vi "interp type 2 1D.vi"(1 "NaN":dbl[](array[numeric]) format="%.2f") -> (0 "Interpolated":dbl[](array[numeric]) format="%.2f")   [LabVIEW 2016, in "comm.lvlib"]
uses:
  comm.lvlib
  <vilib>/Analysis/1siggen.llb/Ramp Pattern by Samples.vi
  <vilib>/Analysis/NI_AALBase.lvlib
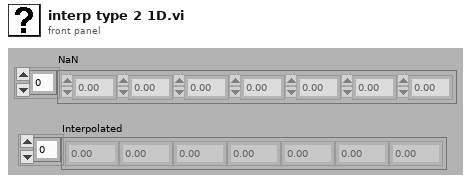
[diagram p1: front panel]
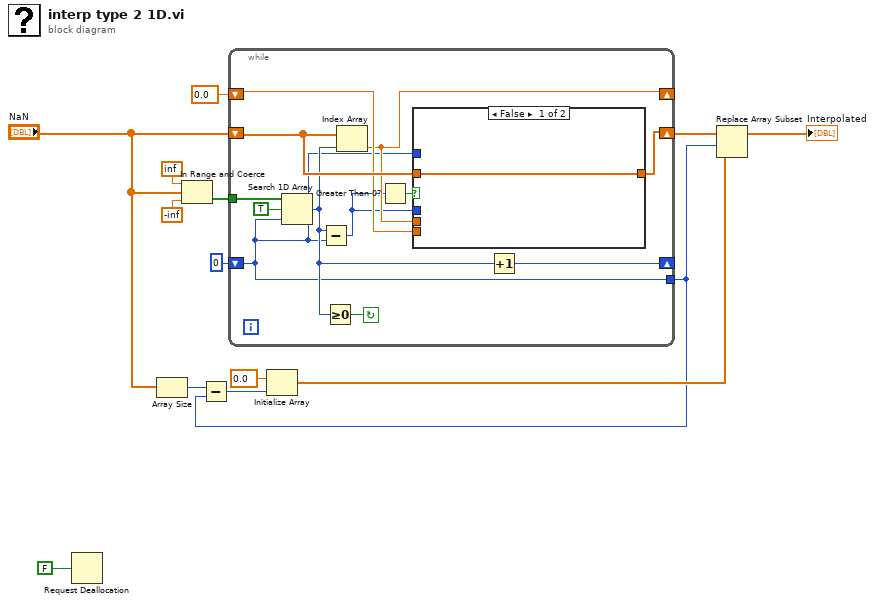
[diagram p0: block diagram]
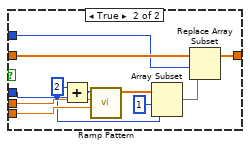
[diagram p2: hidden frame]
diagram:
  n1 = Request Deallocation(FALSE ("flag")) -> ()
  n2 = Array Size(array="NaN") -> (size(s)=w6:i32)
  n3 = In Range and Coerce(upper limit=inf, x="NaN", lower limit=-inf) -> (In Range?=w9:bool[])  [unwired: 1 out]
  n4 = while {
    tunnel: w9 -> [w26]
    shift-right: [w16] -> _
    shift-left: 0 -> [w15]
    shift-right: [w21] -> w3
    shift-left: "NaN" -> [w24]
    shift-right: [w22] -> _
    shift-left: 0.0 ("Numeric") -> [w23]
    tunnel: [w15] -> w1
    stop <- w19 continue-if-true
    n5 = Search 1D Array(1D array=w26, element=TRUE, start index (0)=w15) -> (index of element=w20:i32)
    n6 = Subtract(x=w20, y=w15) -> (x-y=w17:i32)
    n7 = Greater Or Equal To 0?(x=w20) -> (x >= 0?=w19:bool)
    n8 = Index Array(array=w24, index=w20) -> (element=w22:dbl)
    n9 = Greater Than 0?(x=w17) -> (x > 0?=w18:bool)
    n10 = case shown="False" w18 {
      tunnel: w24 -> [w27 w38]
      tunnel: w23 -> [_ w37]
      tunnel: w22 -> [_ w36]
      tunnel: [w27 w35] -> w21
      tunnel: w17 -> [_ w30]
      tunnel: w15 -> [_ w28]
      frame False {
      }
      frame True {
        n11 = Add(x=2, y=w30) -> (x+y=w34:i32)
        n12 = call-poly <vilib>:"Ramp Pattern.vi"("start"=w37, "end"=w36, "samples"=w34) -> ("Ramp Pattern"=w32:dbl[])  [unwired: 7 in, 1 out]
        n13 = Array Subset(array=w32, index=1, length=w30) -> (w29:dbl[])
        n14 = Replace Array Subset(array=w38, new element=w29, index=w28) -> (w35:dbl[])
      }
    }
    n15 = Increment(x=w20) -> (x+1=w16:i32)
  }
  n16 = Subtract(x=w6, y=w1) -> (x-y=w5:i32)
  n17 = Initialize Array(0.0 ("element"), w5) -> (w2:dbl[])
  n18 = Replace Array Subset(array=w3, new element=w2, index=w1) -> (→"Interpolated":dbl[])
